vi "Test Configuration.vi"   [LabVIEW 2016]
uses:
  <vilib>/Utility/sysdir.llb/System Directory Type.ctl
  <userlib>/_OpenG.lib/numeric/numeric.llb/Random Number Within Range - I32__ogtk.vi
  <vilib>/addons/_JKI Toolkits/Caraya/classes/Assert/Assert Equal Value_Variant.vi
  lvsrc/SMOs/Configuration/Configuration.lvclass
  <vilib>/addons/_JKI Toolkits/Caraya/classes/Assert/Assert.lvclass
  <vilib>/addons/_JKI Toolkits/Caraya/classes/Test/Test.lvclass
types:
  T1 = typedef "System Directory Type.ctl" = i32
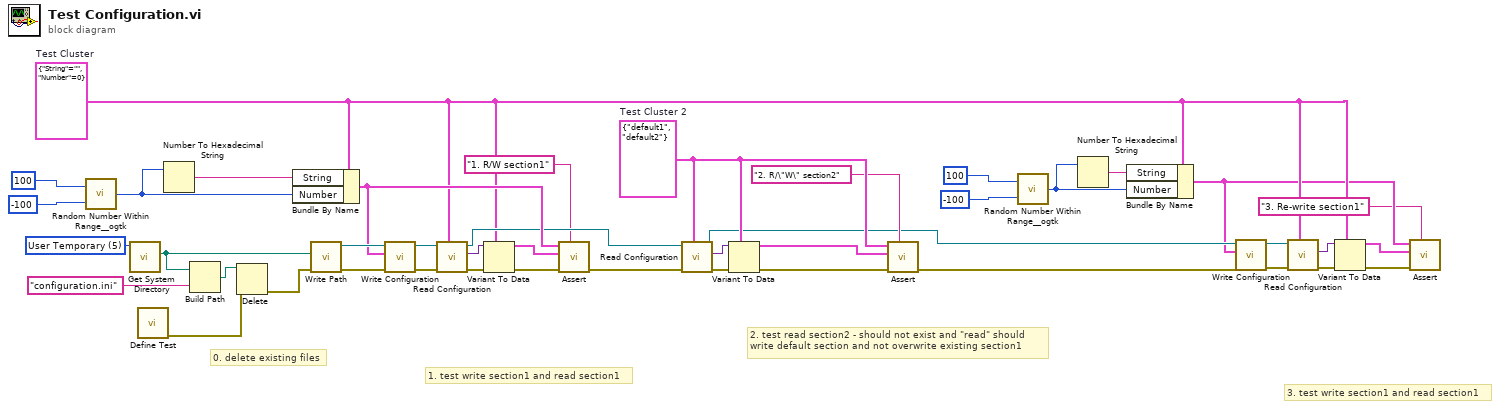
[diagram p0: block diagram]
diagram:
  w23 = cluster{"String":string, "String 2":string} {"String"="default1", "String 2"="default2"}  # Test Cluster 2
  w35 = T1 5 items=["User Home"=0, "User Desktop"=1, "User Documents"=2, "User Application Data"=3, "User Preferences"=4, "User Temporary"=5, "Public Documents"=6, "Public Application Data"=7, "Public Preferences"=8, "Public Cache"=13, "System Core Libraries"=9, "System Installed Libraries"=10, "Application Files"=11, "Boot Volume Root"=12] ("system directory type")
  w3 = cluster{"String":string, "Number":i32} {"String"="", "Number"=0}  # Test Cluster
  # "3. test write section1 and read section1"
  # "0. delete existing files"
  # "2. test read section2 - should not exist and \"read\" should\nwrite default section and not overwrite existing section1"
  # "1. test write section1 and read section1"
  n1 = call-poly <userlib>:"Random Number Within Range__ogtk.vi"("High"=100 ("Number"), "Low"=-100 ("Number")) -> ("Random Number"=w36:i32)  [unwired: 3 in]
  n2 = call <vilib>:"Get System Directory.vi"("system directory type"=w35) -> ("system directory"=w16:path)  [unwired: 10 in]
  n3 = call <vilib>:"Define Test.vi"() -> ("error out"=w18:errorcluster)  [unwired: 11 in]
  n4 = Number To Hexadecimal String(2:w36) -> (0:w37:string)  [unwired: 1 in]
  n5 = Build Path(base path=w16, name or relative path="configuration.ini") -> (appended path=w19:path)
  n6 = Delete(path (use dialog)=w19, error in=w18) -> (error out=w17:errorcluster)  [unwired: 3 in, 2 out]
  n7 = Bundle By Name(cluster=w3, "String"=w37, "Number"=w36) -> (w30:cluster{"String":string, "Number":i32})
  n8 = call "Write Path.vi"("error in (no error)"=w17, "Path"=w16) -> ("error out"=w32:errorcluster, "Configuration out"=w43:refnum<class "Configuration.lvclass">)  [unwired: 8 in]
  n9 = call "Write Configuration.vi"("error in (no error)"=w32, "Variant"=w30, "Configuration in"=w43) -> ("error out"=w40:errorcluster, "Configuration out"=w41:refnum<class "Configuration.lvclass">)  [unwired: 7 in]
  n10 = call "Read Configuration.vi"("INI Fomatted Cluster Type"=w3, "error in (no error)"=w40, "Configuration in"=w41) -> ("error out"=w42:errorcluster, "Configuration"=w34:variant, "Configuration out"=w28:refnum<class "Configuration.lvclass">)  [unwired: 6 in]
  n11 = Variant To Data(error in=w42, type=w3, Variant=w34) -> (data=w31:cluster{"String":string, "Number":i32}, error out=w33:errorcluster)
  n12 = call-poly <vilib>:"Assert.vi"("Label"="1. R/W section1", "error in (no error)"=w33, "Y"=w31, "X"=w30) -> ("error out"=w29:errorcluster)  [unwired: 7 in]
  n13 = call "Read Configuration.vi"("INI Fomatted Cluster Type"=w23, "error in (no error)"=w29, "Configuration in"=w28) -> ("error out"=w27:errorcluster, "Configuration"=w26:variant, "Configuration out"=w7:refnum<class "Configuration.lvclass">)  [unwired: 6 in]
  n14 = Variant To Data(error in=w27, type=w23, Variant=w26) -> (data=w24:cluster{"String":string, "String 2":string}, error out=w25:errorcluster)
  n15 = call-poly <vilib>:"Assert.vi"("Label"="2. R/\"W\" section2", "error in (no error)"=w25, "Y"=w24, "X"=w23) -> ("error out"=w12:errorcluster)  [unwired: 7 in]
  n16 = call-poly <userlib>:"Random Number Within Range__ogtk.vi"("High"=100 ("Number"), "Low"=-100 ("Number")) -> ("Random Number"=w11:i32)  [unwired: 3 in]
  n17 = Number To Hexadecimal String(2:w11) -> (0:w10:string)  [unwired: 1 in]
  n18 = Bundle By Name(cluster=w3, "String"=w10, "Number"=w11) -> (w2:cluster{"String":string, "Number":i32})
  n19 = call "Write Configuration.vi"("error in (no error)"=w12, "Variant"=w2, "Configuration in"=w7) -> ("error out"=w14:errorcluster, "Configuration out"=w5:refnum<class "Configuration.lvclass">)  [unwired: 7 in]
  n20 = call "Read Configuration.vi"("INI Fomatted Cluster Type"=w3, "error in (no error)"=w14, "Configuration in"=w5) -> ("error out"=w13:errorcluster, "Configuration"=w6:variant)  [unwired: 6 in, 1 out]
  n21 = Variant To Data(error in=w13, type=w3, Variant=w6) -> (data=w4:cluster{"String":string, "Number":i32}, error out=w15:errorcluster)
  n22 = call-poly <vilib>:"Assert.vi"("Label"="3. Re-write section1", "error in (no error)"=w15, "Y"=w4, "X"=w2) -> ()  [unwired: 7 in, 1 out]
